vi "Initiate Updates.vi"(8 "error in (no error)":errorcluster, 11 "IViewable In":refnum<class "IViewable.lvclass">) -> (0 "error out":errorcluster, 3 "IViewable Out":refnum<class "IViewable.lvclass">)   [LabVIEW 2020, in "IViewable.lvlib" / "IViewable.lvclass"]
doc: "初始化更新"
uses:
  IViewable.lvclass
  IViewable.lvclass/IViewable.ctl
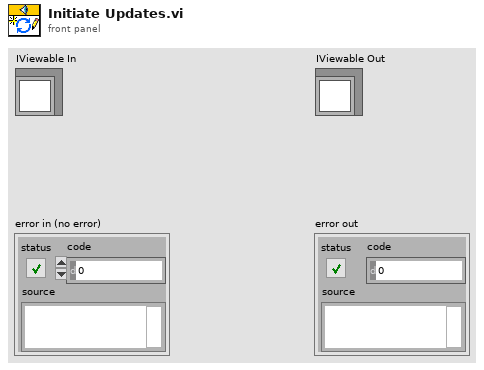
[diagram p1: front panel]
types:
  T1 = enum32{"Invalid", "Standard", "Closed", "Hidden", "Minimized", "Maximized"}
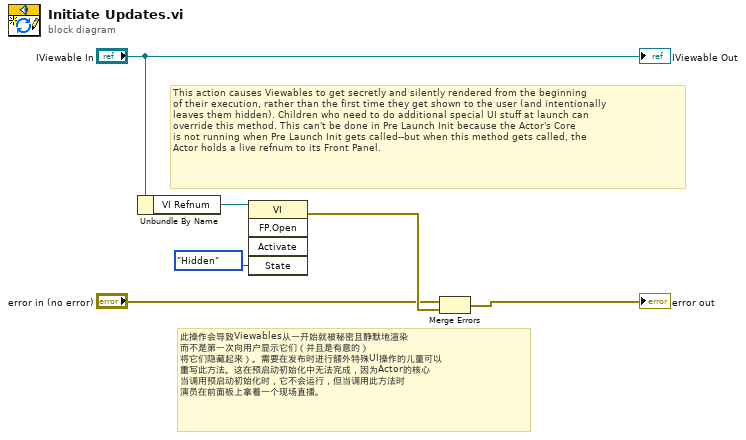
[diagram p0: block diagram]
diagram:
  # "此操作会导致Viewables从一开始就被秘密且静默地渲染\n而不是第一次向用户显示它们（并且是有意的）\n将它们隐藏起来）。需要在发布时进行额外特殊UI操作的儿童可以\n重写此方法。这在预启动初始化中无法完成，因为Actor的核心\n当调用预启动初始化时，它不会运行，但当调用此方法时\n演员在前面板上拿着一个现场直播。"
  # "This action causes Viewables to get secretly and silently rendered from the beginning\nof their execution, rather than the first time they get shown to the user (and intentionally\nleaves them hidden). Children who need to do additional special UI stuff at launch can\noverride this method. This can't be done in Pre Launch Init because the Actor's Core\nis not running when Pre Launch Init gets called--but when this method gets called, the\nActor holds a live refnum to its Front Panel."
  n1 = Unbundle By Name("IViewable In") -> ("VI Refnum"=w1:refnum<vi>)
  n2 = invoke class="VI" method="FP.Open"(reference=w1, "State"=T1."Hidden") -> (error out=w6:errorcluster)  [unwired: 3 in, 4 out]
  n3 = Merge Errors("error in (no error)", w6) -> (→"error out":errorcluster)
  "IViewable Out" <- "IViewable In"
